vi "SetJogAcceleration.vi"(8 "Error In":errorcluster, 10 "Jog Acceleration":dbl, 11 "Thorlabs In":refnum<class "Thorlabs.lvclass">) -> (0 "Error Out":errorcluster, 3 "Thorlabs Out":refnum<class "Thorlabs.lvclass">)   [LabVIEW 2018, in "Thorlabs.lvlib" / "Thorlabs.lvclass"]
doc: "This VI sets the job acceleration on the Axis.\n\nCreator: Slade Jeppesen\nCreated Date: 10/02/20"
uses:
  Thorlabs.lvclass
  Thorlabs.lvclass/Thorlabs.ctl
  C:/AME Test Engineering/LabVIEW/PPLs/Axis/DLLs/ThorLabs.MotionControl.KCube.DCServoCLI.dll
  PPLs/Axis/DLLs/ThorLabs.MotionControl.KCube.DCServoCLI.dll
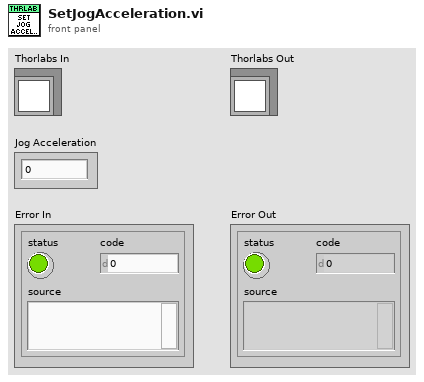
[diagram p1: front panel]
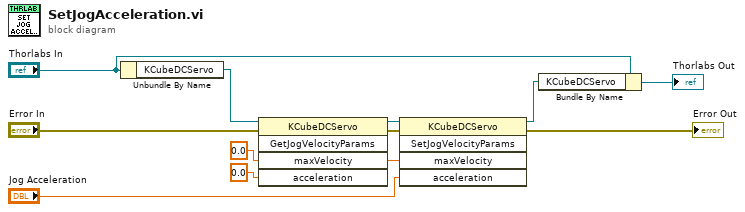
[diagram p0: block diagram]
diagram:
  n1 = Unbundle By Name("Thorlabs In") -> ("KCubeDCServo"=w12:refnum<k24>)
  n2 = invoke class="KCubeDCServo" method="GetJogVelocityParams"(reference=w12, error in="Error In", "maxVelocity"=0.0, "acceleration"=0.0) -> (reference out=w8:refnum<k24>, error out=w1:errorcluster, "maxVelocity"=w5:dbl)  [unwired: 1 in, 2 out]
  n3 = invoke class="KCubeDCServo" method="SetJogVelocityParams"(reference=w8, error in=w1, "maxVelocity"=w5, "acceleration"="Jog Acceleration") -> (reference out=w7:refnum<k24>, error out=→"Error Out":errorcluster)  [unwired: 1 in, 3 out]
  n4 = Bundle By Name(cluster="Thorlabs In", "KCubeDCServo"=w7) -> (→"Thorlabs Out":refnum<class "Thorlabs.lvclass">)
